vi "Update UI.vi"(8 "error in (no error)":errorcluster, 10 "DataExchange":T1, 11 "StepMotorController in":refnum<class "StepMotorController.lvclass">) -> (0 "error out":errorcluster, 3 "StepMotorController out":refnum<class "StepMotorController.lvclass">)   [LabVIEW 2020, in "StepMotorController.lvlib" / "StepMotorController.lvclass"]
uses:
  StepMotorController.lvclass
  Model/Hardware Abstraction Layer/Component/Device/Device/DataExchange.ctl
  StepMotorController.lvclass/StepMotorController.ctl
  Interface/DataListener/DataListener.lvclass
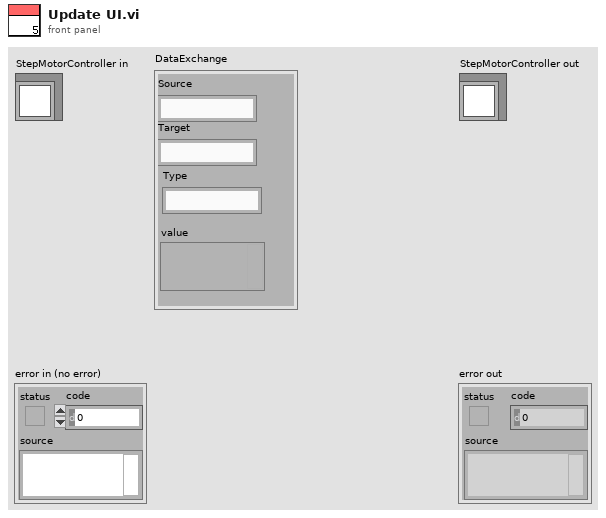
[diagram p1: front panel]
types:
  T1 = typedef "DataListener.lvclass/DataExchange.ctl" = cluster{"Source":string, "Target":string, "Type":string, "value":variant}
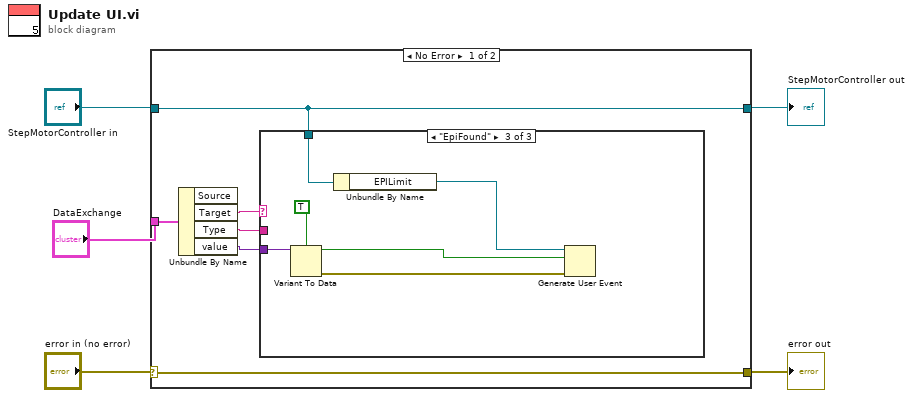
[diagram p0: block diagram]
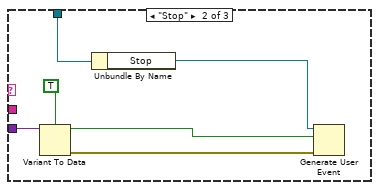
[diagram p3: hidden frame]
diagram:
  n1 = case shown="No Error" "error in (no error)" {
    selector: "error in (no error)" -> [w11 w25]
    tunnel: [w11 w25] -> w1
    tunnel: [w6 w24] -> w2
    tunnel: "StepMotorController in" -> [w6 w24]
    tunnel: "DataExchange" -> [w10 _]
    frame No Error {
      n2 = Unbundle By Name(w10) -> ("Target"=w7:string, "Type"=w8:string, "value"=w9:variant)  [unwired: 1 out]
      n3 = case shown="\"EpiFound\"" w7 {
        tunnel: w9 -> [_ w17 w23]
        tunnel: w8 -> [_ _ _]
        tunnel: w6 -> [_ w16 w22]
        frame "False", Default {
        }
        frame "Stop" {
          n4 = Variant To Data(type=TRUE, Variant=w17) -> (data=w14:bool, error out=w12:errorcluster)  [unwired: 1 in]
          n5 = Unbundle By Name(w16) -> ("Stop"=w15:refnum<user-event>)
          n6 = Generate User Event(user event=w15, event data cluster=w14, error in=w12) -> ()  [unwired: 1 in, 2 out]
        }
        frame "EpiFound" {
          n7 = Variant To Data(type=TRUE, Variant=w23) -> (data=w20:bool, error out=w18:errorcluster)  [unwired: 1 in]
          n8 = Unbundle By Name(w22) -> ("EPILimit"=w21:refnum<user-event>)
          n9 = Generate User Event(user event=w21, event data cluster=w20, error in=w18) -> ()  [unwired: 1 in, 2 out]
        }
      }
    }
    frame Error {
    }
  }
  "error out" <- w1
  "StepMotorController out" <- w2
